vi "TIO SLIP Serial Write.vi"(8 "error in (no error)":errorcluster, 10 "Data":string, 11 "VISA Refnum in":refnum<visa-resource-name>) -> (0 "error out":errorcluster)   [LabVIEW 2017]
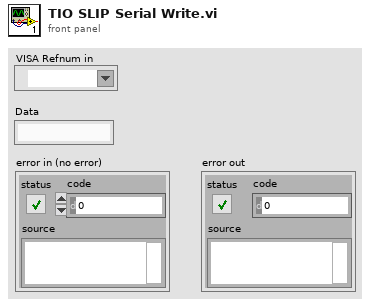
[diagram p1: front panel]
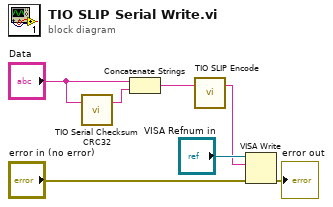
[diagram p0: block diagram]
diagram:
  n1 = call "TIO Serial Checksum CRC32.vi"("String"="Data") -> ("CRC32 Little Endian String"=w3:string)  [unwired: 1 in, 1 out]
  n2 = Concatenate Strings("Data", w3) -> (w2:string)
  n3 = call "TIO SLIP Encode.vi"("String Input"=w2) -> ("SLIP Output"=w5:string)  [unwired: 1 in, 1 out]
  n4 = VISA Write(VISA resource name="VISA Refnum in", write buffer=w5, error in (no error)="error in (no error)") -> (error out=→"error out":errorcluster)  [unwired: 2 out]
